vi "DAQ EVENTS.vi"() -> ()   [LabVIEW 2018]
panel:
  in  "Enum":T1(ring)
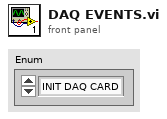
[diagram p1: front panel]
types:
  T1 = enum16{"INIT DAQ CARD", "SET HV ON CHANNELTRON", "SET FEMTO GAIN"}
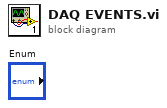
[diagram p0: block diagram]
diagram:
